vi "GOOP_CropImage.vi"(4 "subset rect":T1, 6 "image data":T2) -> (0 "true subset rect":T1, 2 "image subset":T2)   [LabVIEW 2016]
doc: "Returns a subset of a source image instead of the entire image. Use the Picture to Pixmap VI to convert a picture to a cluster you can wire to <B>image data</B>."
uses:
  <vilib>/picture/picture.llb/imagedata.ctl
panel:
  out "2D Picture 2":picture
  out "2D Picture":picture
  out "mask":u8[](array[numeric]) format="%08b"
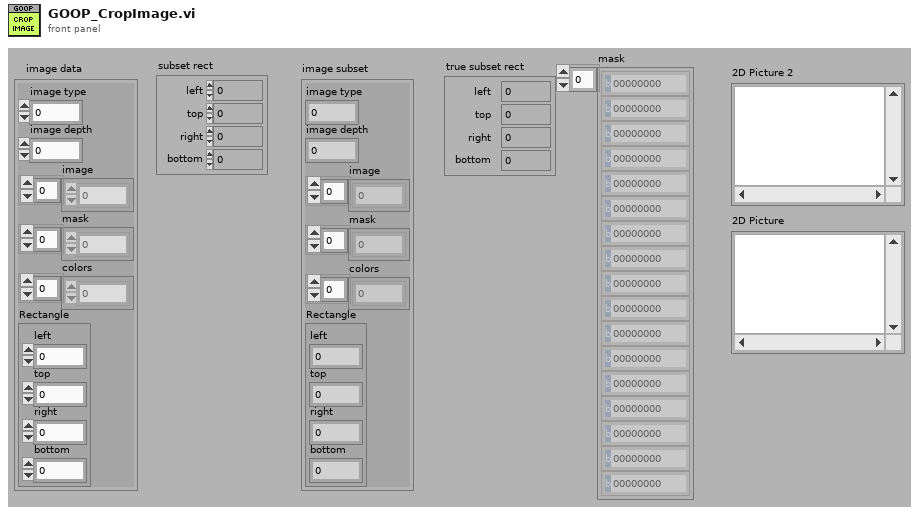
[diagram p1: front panel]
types:
  T1 = cluster{"left":i16, "top":i16, "right":i16, "bottom":i16}
  T2 = typedef "imagedata.ctl" = cluster{"image type":i32, "image depth":i32, "image":u8[], "mask":u8[], "colors":u32[], "Rectangle":cluster{"left":i16, "top":i16, "right":i16, "bottom":i16}}
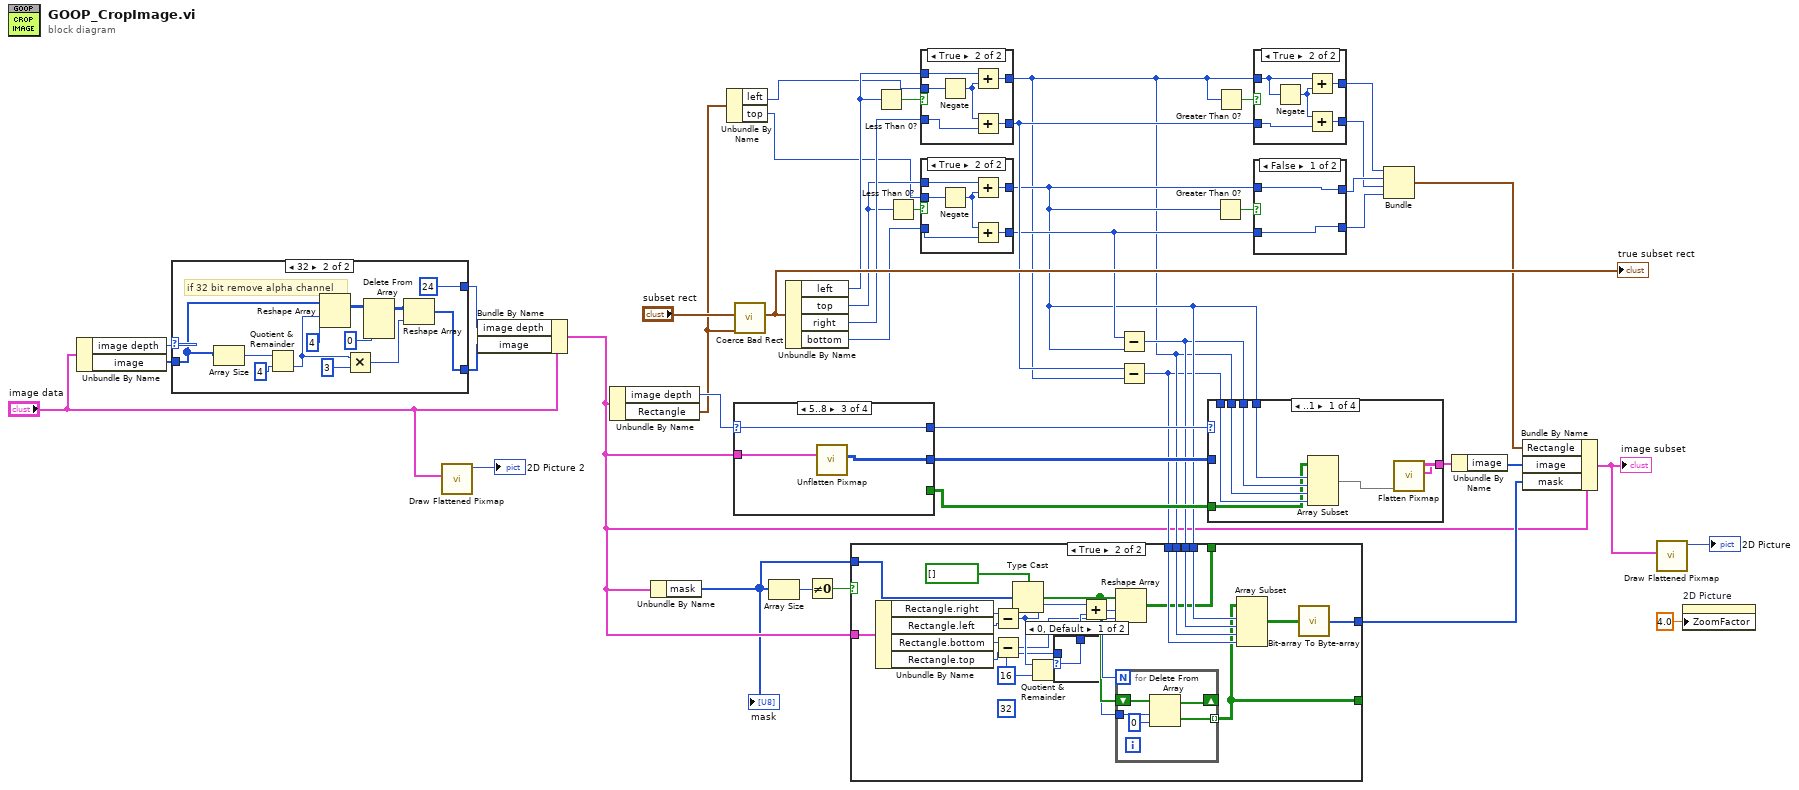
[diagram p0: block diagram]
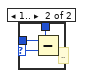
[diagram p3: hidden frame]
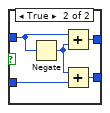
[diagram p5: hidden frame]
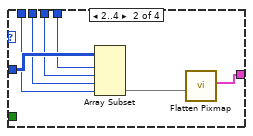
[diagram p9: hidden frame]
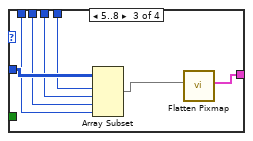
[diagram p10: hidden frame]
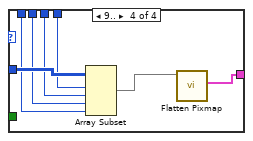
[diagram p11: hidden frame]
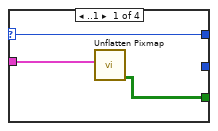
[diagram p12: hidden frame]
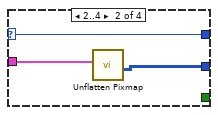
[diagram p13: hidden frame]
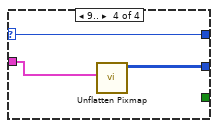
[diagram p14: hidden frame]
diagram:
  n1 = Unbundle By Name("image data") -> ("image depth"=w20:i32, "image"=w19:u8[])
  n2 = case shown="32" w20 {
    selector: w20 -> [w46 _]
    tunnel: [w46 24] -> w18
    tunnel: w19 -> [w45 w57]
    tunnel: [w45 w48] -> w17
    frame 1, 2, 4, 8, 24, Default {
    }
    frame 32 {
      # "if 32 bit remove alpha channel"
      n3 = Array Size(array=w57) -> (size(s)=w56:i32)
      n4 = Quotient & Remainder(x=w56, y=4) -> (floor(x/y)=w52:i32)  [unwired: 1 out]
      n5 = Reshape Array(w57, w52, 4 ("dimension size")) -> (w54:u8[][])
      n6 = Multiply(x=w52, y=3) -> (x*y=w50:i32)
      n7 = Delete From Array(array=w54, index (col)=0 ("dimension size")) -> (array with subset deleted=w49:u8[][])  [unwired: 2 in, 1 out]
      n8 = Reshape Array(w49, w50) -> (w48:u8[])
    }
  }
  n9 = call <vilib>:"Draw Flattened Pixmap.vi"("image data"="image data") -> ("new picture"=→"2D Picture 2":picture)  [unwired: 8 in]
  n10 = Bundle By Name(cluster="image data", "image depth"=w18, "image"=w17) -> (w9:T2)
  n11 = Unbundle By Name(w9) -> ("image depth"=w42:i32, "Rectangle"=w23:T1)
  n12 = Unbundle By Name(w9) -> ("mask"=w6:u8[])
  "mask" <- w6
  n13 = Unbundle By Name(w23) -> ("left"=w22:i16, "top"=w21:i16)
  n14 = case shown="5..8" w42 {
    selector: w42 -> [w61 w64 w67 w68]
    tunnel: [_ w63 w66 w70] -> w43
    tunnel: [w60 _ _ _] -> w44
    tunnel: [w61 w64 w67 w68] -> w40
    tunnel: w9 -> [w59 w62 w65 w69]
    frame ..1 {
      n15 = call <vilib>:"Unflatten Pixmap.vi"("image data"=w59) -> ("1-bit pixmap"=w60:bool[][])  [unwired: 4 in, 6 out]
    }
    frame 2..4 {
      n16 = call <vilib>:"Unflatten Pixmap.vi"("image data"=w62) -> ("4-bit pixmap"=w63:u8[][])  [unwired: 4 in, 6 out]
    }
    frame 5..8 {
      n17 = call <vilib>:"Unflatten Pixmap.vi"("image data"=w65) -> ("8-bit pixmap"=w66:u8[][])  [unwired: 4 in, 6 out]
    }
    frame 9.. {
      n18 = call <vilib>:"Unflatten Pixmap.vi"("image data"=w69) -> ("24-bit pixmap"=w70:u32[][])  [unwired: 4 in, 6 out]
    }
  }
  n19 = call <vilib>:"Coerce Bad Rect.vi"("image rect"=w23, "subset rect"="subset rect") -> ("Rectangle"=w38:T1)  [unwired: 9 in]
  "true subset rect" <- w38
  n20 = Array Size(array=w6) -> (size(s)=w8:i32)
  n21 = Unbundle By Name(w38) -> ("left"=w35:i16, "top"=w33:i16, "right"=w36:i16, "bottom"=w32:i16)
  n22 = Not Equal To 0?(x=w8) -> (x != 0?=w7:bool)
  n23 = Less Than 0?(x=w35) -> (x < 0?=w37:bool)
  n24 = Less Than 0?(x=w33) -> (x < 0?=w34:bool)
  n25 = case shown="True" w37 {
    tunnel: w35 -> [w72 w74]
    tunnel: w36 -> [w71 w75]
    tunnel: [w72 w78] -> w14
    tunnel: [w71 w76] -> w30
    tunnel: w22 -> [_ w73]
    frame False {
    }
    frame True {
      n26 = Negate(x=w73) -> (-x=w77:i16)
      n27 = Add(x=w74, y=w77) -> (x+y=w78:i16)
      n28 = Add(x=w77, y=w75) -> (x+y=w76:i16)
    }
  }
  n29 = case shown="True" w34 {
    tunnel: w33 -> [w80 w82]
    tunnel: w32 -> [w79 w84]
    tunnel: [w80 w86] -> w16
    tunnel: [w79 w83] -> w28
    tunnel: w21 -> [_ w81]
    frame False {
    }
    frame True {
      n30 = Negate(x=w81) -> (-x=w85:i16)
      n31 = Add(x=w82, y=w85) -> (x+y=w86:i16)
      n32 = Add(x=w85, y=w84) -> (x+y=w83:i16)
    }
  }
  n33 = Subtract(x=w28, y=w16) -> (x-y=w15:i16)
  n34 = Subtract(x=w30, y=w14) -> (x-y=w13:i16)
  n35 = case shown="True" w7 {
    tunnel: w16 -> [_ w104]
    tunnel: w15 -> [_ w103]
    tunnel: w14 -> [_ w102]
    tunnel: w13 -> [_ w101]
    tunnel: [w87 w99] -> w12
    tunnel: w9 -> [_ w98]
    tunnel: w6 -> [w87 w97]
    tunnel: [_ w88] -> _
    tunnel: [_ w89] -> _
    frame False {
    }
    frame True {
      (unwired) i16 32 ("y")
      w93 = i16 16 ("y")
      n36 = Unbundle By Name(w98) -> ("Rectangle.right"=w108:i16, "Rectangle.left"=w107:i16, "Rectangle.bottom"=w106:i16, "Rectangle.top"=w105:i16)
      n37 = Subtract(x=w108, y=w107) -> (x-y=w96:i16)
      n38 = Subtract(x=w106, y=w105) -> (x-y=w92:i16)
      n39 = Type Cast(type=bool[] [], x=w97) -> (*(type *) &x=w91:bool[])
      n40 = Quotient & Remainder(x=w96, y=w93) -> (x-y*floor(x/y)=w95:i16)  [unwired: 1 out]
      n41 = case shown="0, Default" w95 {
        selector: w95 -> [w110 w113]
        tunnel: [w110 w112] -> w94
        tunnel: w93 -> [_ w111]
        frame 0, Default {
        }
        frame 1.. {
          # ".."
          n42 = Subtract(x=w111, y=w113) -> (x-y=w112:i16)
        }
      }
      n43 = Add(x=w96, y=w94) -> (x+y=w90:i16)
      n44 = Reshape Array(w91, w90, w92) -> (w89:bool[][])
      n45 = for {
        N: w92 -> [_]
        shift-right: [w117] -> _
        shift-left: w91 -> [w118]
        tunnel: w90 -> [w115]
        tunnel: [w114] -> w88 mode=indexing
        n46 = Delete From Array(array=w118, length=w115, index=0) -> (deleted portion=w114:bool[], array with subset deleted=w117:bool[])
      }
      n47 = Array Subset(array=w88, index (row)=w104, length (row)=w103, index (col)=w102, length (col)=w101) -> (w100:bool[][])
      n48 = call <vilib>:"Bit-array To Byte-array.vi"("bit array"=w100) -> ("byte array"=w99:u8[])
    }
  }
  n49 = case shown="..1" w40 {
    tunnel: w43 -> [_ w131 w139 w146]
    tunnel: w44 -> [w119 _ _ _]
    tunnel: w16 -> [w125 w129 w136 w143]
    tunnel: w15 -> [w124 w127 w134 w141]
    tunnel: w14 -> [w123 w128 w135 w142]
    tunnel: w13 -> [w122 w126 w133 w140]
    tunnel: [w120 w130 w137 w144] -> w41
    frame ..1 {
      n50 = Array Subset(array=w119, index (row)=w125, length (row)=w124, index (col)=w123, length (col)=w122) -> (w121:bool[][])
      n51 = call <vilib>:"Flatten Pixmap.vi"("1-bit pixmap"=w121) -> ("image data"=w120:T2)  [unwired: 10 in]
    }
    frame 2..4 {
      n52 = Array Subset(array=w131, index (row)=w129, length (row)=w127, index (col)=w128, length (col)=w126) -> (w132:u32[][])
      n53 = call <vilib>:"Flatten Pixmap.vi"("4-bit pixmap"=w132) -> ("image data"=w130:T2)  [unwired: 10 in]
    }
    frame 5..8 {
      n54 = Array Subset(array=w139, index (row)=w136, length (row)=w134, index (col)=w135, length (col)=w133) -> (w138:u32[][])
      n55 = call <vilib>:"Flatten Pixmap.vi"("8-bit pixmap"=w138) -> ("image data"=w137:T2)  [unwired: 10 in]
    }
    frame 9.. {
      n56 = Array Subset(array=w146, index (row)=w143, length (row)=w141, index (col)=w142, length (col)=w140) -> (w145:u32[][])
      n57 = call <vilib>:"Flatten Pixmap.vi"("24-bit pixmap"=w145) -> ("image data"=w144:T2)  [unwired: 10 in]
    }
  }
  n58 = Greater Than 0?(x=w16) -> (x > 0?=w29:bool)
  n59 = Greater Than 0?(x=w14) -> (x > 0?=w31:bool)
  n60 = case shown="True" w31 {
    tunnel: w14 -> [w148 w153]
    tunnel: w30 -> [w147 w151]
    tunnel: [w148 w150] -> w27
    tunnel: [w147 w149] -> w25
    frame False {
    }
    frame True {
      n61 = Negate(x=w153) -> (-x=w152:i16)
      n62 = Add(x=w153, y=w152) -> (x+y=w150:i16)
      n63 = Add(x=w152, y=w151) -> (x+y=w149:i16)
    }
  }
  n64 = case shown="False" w29 {
    tunnel: w16 -> [w155 w159]
    tunnel: w28 -> [w154 w158]
    tunnel: [w155 w157] -> w26
    tunnel: [w154 w156] -> w24
    frame False {
    }
    frame True {
      n65 = Negate(x=w159) -> (-x=w160:i16)
      n66 = Add(x=w159, y=w160) -> (x+y=w157:i16)
      n67 = Add(x=w160, y=w158) -> (x+y=w156:i16)
    }
  }
  n68 = Bundle("left"=w27, "top"=w26, "right"=w25, "bottom"=w24) -> (w11:T1)  [unwired: 1 in]
  n69 = Unbundle By Name(w41) -> ("image"=w10:u8[])
  n70 = Bundle By Name(cluster=w9, "Rectangle"=w11, "image"=w10, "mask"=w12) -> (w3:T2)
  "image subset" <- w3
  n71 = call <vilib>:"Draw Flattened Pixmap.vi"("image data"=w3) -> ("new picture"=→"2D Picture":picture)  [unwired: 8 in]
  n72 = property on="2D Picture" class="Pict"("ZoomFactor"=sgl 4.0 ("Zoom Factor")) -> ()  [unwired: 2 in, 2 out]
